vi "PSSTRING_Check Double Quotation Marks.vi"(10 "String":string) -> (1 "\"Tag\"[]":string[](array[string]), 2 "Error?":bool)   [LabVIEW 2016]
uses:
  <vilib>/regexp/Match Regular Expression.xnode
panel:
  # "Data In"
  # "Data Out"
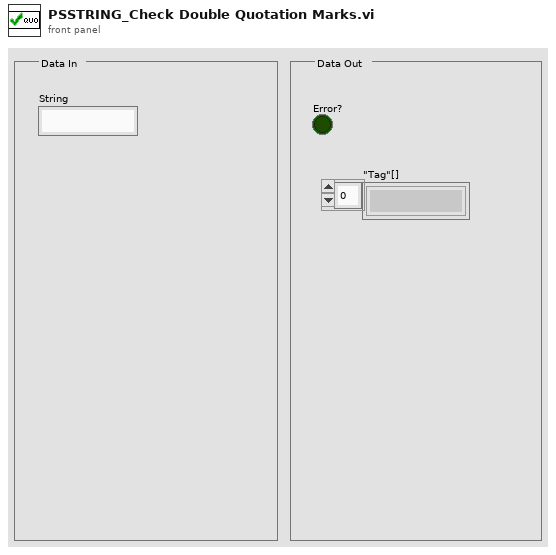
[diagram p1: front panel]
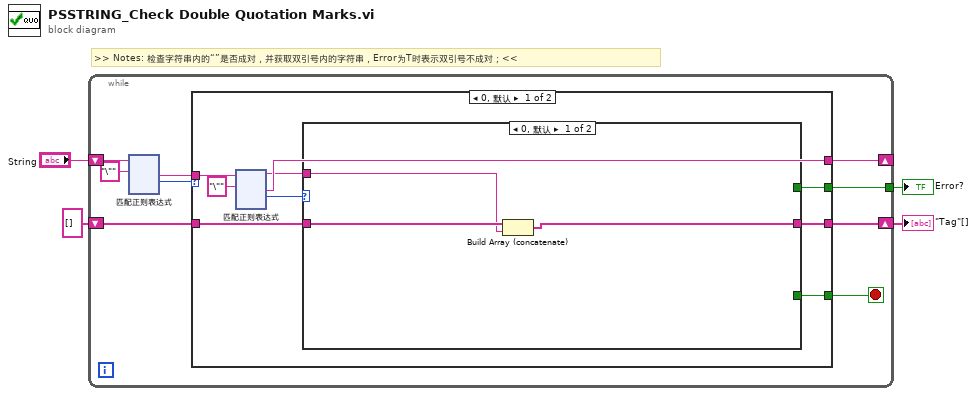
[diagram p0: block diagram]
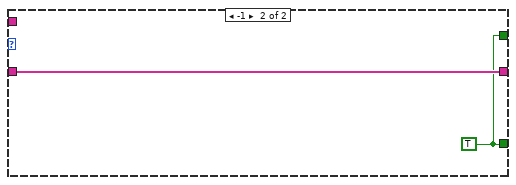
[diagram p2: hidden frame]
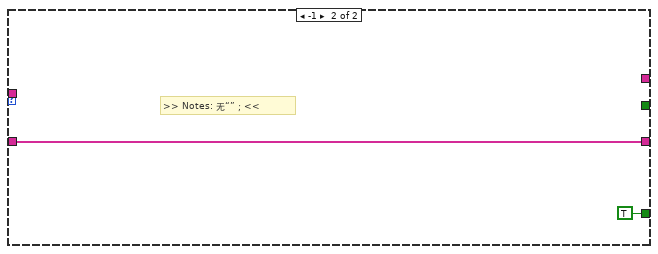
[diagram p3: hidden frame]
diagram:
  # ">> Notes: 检查字符串内的“”是否成对，并获取双引号内的字符串，Error为T时表示双引号不成对；<<"
  n1 = while {
    shift-right: [w9] -> _
    shift-left: "String" -> [w13]
    shift-right: [w6] -> w2
    shift-left: string[] [] -> [w7]
    tunnel: [w5] -> w1
    stop <- w8 stop-if-true
    n2 = xnode "匹配正则表达式"("输入字符串"=w13, "正则表达式"="\"") -> ("匹配之后"=w10:string, "匹配后偏移量"=w11:i32)  [unwired: 4 in, 3 out]
    n3 = case shown="0, 默认" w11 {
      tunnel: w10 -> [w21 _]
      tunnel: [w19 _] -> w9
      tunnel: [w17 TRUE] -> w8
      tunnel: w7 -> [w16 w143]
      tunnel: [w15 w143] -> w6
      tunnel: [w14 _] -> w5
      frame 0, Default {
        n4 = xnode "匹配正则表达式"("输入字符串"=w21, "正则表达式"="\"") -> ("匹配之前"=w18:string, "匹配之后"=w19:string, "匹配后偏移量"=w20:i32)  [unwired: 4 in, 2 out]
        n5 = case shown="0, 默认" w20 {
          tunnel: w18 -> [w24 _]
          tunnel: [_ w26] -> w17
          tunnel: w16 -> [w25 w27]
          tunnel: [w23 w27] -> w15
          tunnel: [_ w26] -> w14
          frame 0, Default {
            n6 = Build Array (concatenate)(w25, w24) -> (w23:string[])
          }
          frame -1 {
            w26 = TRUE
          }
        }
      }
      frame -1 {
        # ">> Notes: 无“”；<<"
      }
    }
  }
  "\"Tag\"[]" <- w2
  "Error?" <- w1
